vi "Scale_RT Host.vi"(10 "Number of Teeth in Sensor":dbl=2.0, 11 "Tach Period (uSec/pulse)":u32) -> (3 "RPM":dbl)   [LabVIEW 2012]
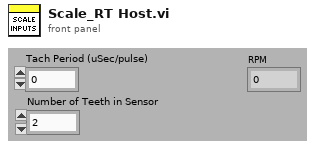
[diagram p1: front panel]
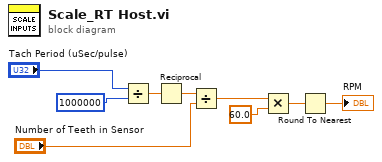
[diagram p0: block diagram]
diagram:
  n1 = Divide(x="Tach Period (uSec/pulse)", y=u32 1000000) -> (x/y=w8:dbl)
  n2 = Reciprocal(x=w8) -> (1/x=w3:dbl)
  n3 = Divide(x=w3, y="Number of Teeth in Sensor") -> (x/y=w2:dbl)
  n4 = Multiply(x=w2, y=60.0) -> (x*y=w5:dbl)
  n5 = Round To Nearest(number=w5) -> (nearest integer value=→"RPM":dbl)
